vi "Set Active Channel.vi"(8 "error in":errorcluster, 11 "3300 in":refnum<class "3300.lvclass">) -> (0 "error out":errorcluster, 3 "3300 out":refnum<class "3300.lvclass">)   [LabVIEW 2019, in "3300.lvlib" / "3300.lvclass"]
uses:
  Library/3300.lvclass
  C:/Users/Public/Documents/Development/builds/Instruments/Electronic Load.lvlibp/Library/Electronic Load.lvclass
  Library/3300.lvclass/3300.ctl
  Accessors/Read Local Resource.vi
  Accessors/Write Local Resource.vi
  builds/Instruments/Electronic Load.lvlibp/Accessors/Read Active Channel.vi
  <instrlib>/Agilent N330X Series/Agilent N330X Series.lvlib
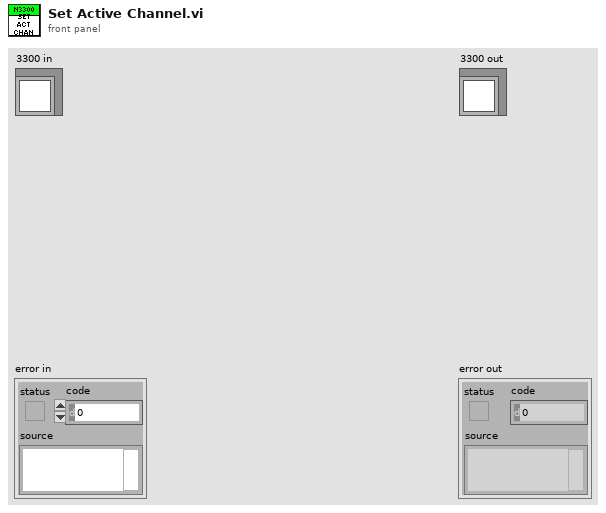
[diagram p1: front panel]
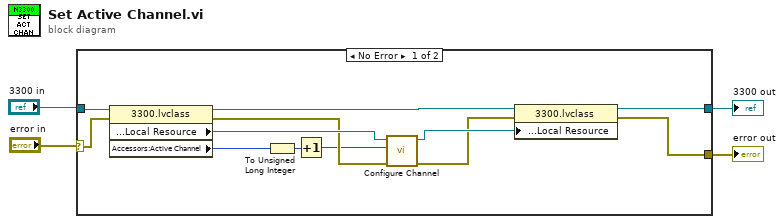
[diagram p0: block diagram]
diagram:
  n1 = case shown="No Error" "error in" {
    selector: "error in" -> [w9 w18]
    tunnel: [w8 w18] -> w3
    tunnel: [w12 w17] -> w1
    tunnel: "3300 in" -> [w16 w17]
    frame No Error {
      n2 = property class="3300.lvclass"(reference=w16, error in=w9) -> (reference out=w13:refnum<class "3300.lvclass">, error out=w14:errorcluster, "Private:Accessors:Local Resource"=w15:refnum<visa-resource-name>, "Accessors:Active Channel"=w5:u32)
      n3 = To Unsigned Long Integer(number=w5) -> (unsigned 32bit integer=w7:u32)
      n4 = Increment(x=w7) -> (x+1=w6:u32)
      n5 = call <instrlib>:"Configure Channel.vi"("error in (no error)"=w14, "Channel (1)"=w6, "VISA resource name"=w15) -> ("error out"=w10:errorcluster, "VISA resource name out"=w11:refnum<visa-resource-name>)  [unwired: 7 in]
      n6 = property class="3300.lvclass"(reference=w13, error in=w10, "Private:Accessors:Local Resource"=w11) -> (reference out=w12:refnum<class "3300.lvclass">, error out=w8:errorcluster)
    }
    frame Error {
    }
  }
  "error out" <- w3
  "3300 out" <- w1
